vi "Find subSchedule Position.vi"(9 "SubSchedule":refnum<class "Schedule.lvclass">, 10 "initial index":i32, 11 "Schedule in":refnum<class "Schedule.lvclass">) -> (2 "index of subarray":i32, 3 "Schedule out":refnum<class "Schedule.lvclass">)   [LabVIEW 2020, in "Run Utilities.lvlib" / "Schedule.lvclass"]
uses:
  Schedule.lvclass
  Schedule.lvclass/Schedule.ctl
panel:
  out "error out":errorcluster
  in  "error in (no error)":errorcluster
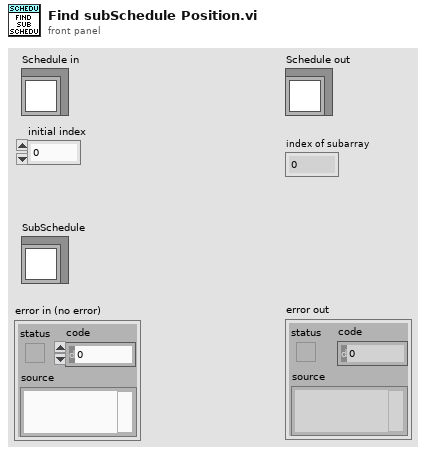
[diagram p1: front panel]
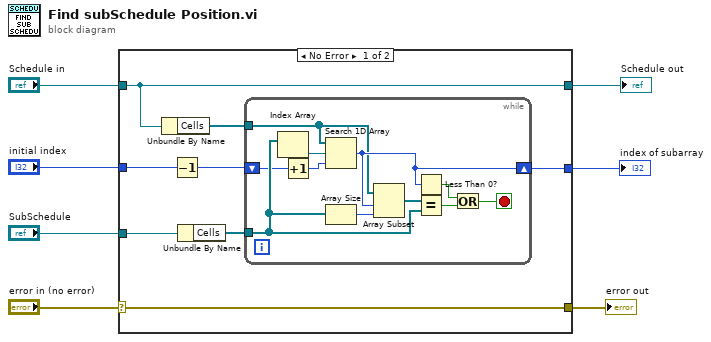
[diagram p0: block diagram]
diagram:
  n1 = case shown="No Error" "error in (no error)" {
    selector: "error in (no error)" -> [w9 w29]
    tunnel: [w15 w28] -> w7
    tunnel: "initial index" -> [w14 w28]
    tunnel: "Schedule in" -> [w8 w27]
    tunnel: "SubSchedule" -> [w12 _]
    tunnel: [w9 w29] -> w2
    tunnel: [w8 w27] -> w1
    frame No Error {
      n2 = Unbundle By Name(w8) -> ("Cells"=w11:refnum<class "Schedule Cell.lvclass">[])
      n3 = Decrement(x=w14) -> (x-1=w13:i32)
      n4 = Unbundle By Name(w12) -> ("Cells"=w10:refnum<class "Schedule Cell.lvclass">[])
      n5 = while {
        tunnel: w11 -> [w16]
        tunnel: w10 -> [w23]
        shift-right: [w19] -> w15
        shift-left: w13 -> [w18]
        stop <- w21 stop-if-true
        n6 = Index Array(array=w23) -> (element=w26:refnum<class "Schedule Cell.lvclass">)  [unwired: 1 in]
        n7 = Increment(x=w18) -> (x+1=w17:i32)
        n8 = Search 1D Array(1D array=w16, element=w26, start index (0)=w17) -> (index of element=w19:i32)
        n9 = Array Size(array=w23) -> (size(s)=w25:i32)
        n10 = Array Subset(array=w16, index=w19, length=w25) -> (w24:refnum<class "Schedule Cell.lvclass">[])
        n11 = Less Than 0?(x=w19) -> (x < 0?=w22:bool)
        n12 = Equal?(x=w24, y=w23) -> (x = y?=w20:bool)
        n13 = Or(x=w22, y=w20) -> (x .or. y?=w21:bool)
      }
    }
    frame Error {
    }
  }
  "index of subarray" <- w7
  "Schedule out" <- w1
  "error out" <- w2
